vi "ReMiRCAutoCamCalibration.vi"() -> ()   [LabVIEW 2019]
panel:
  in  "stop":bool
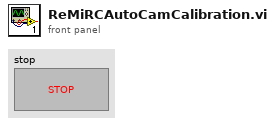
[diagram p1: front panel]
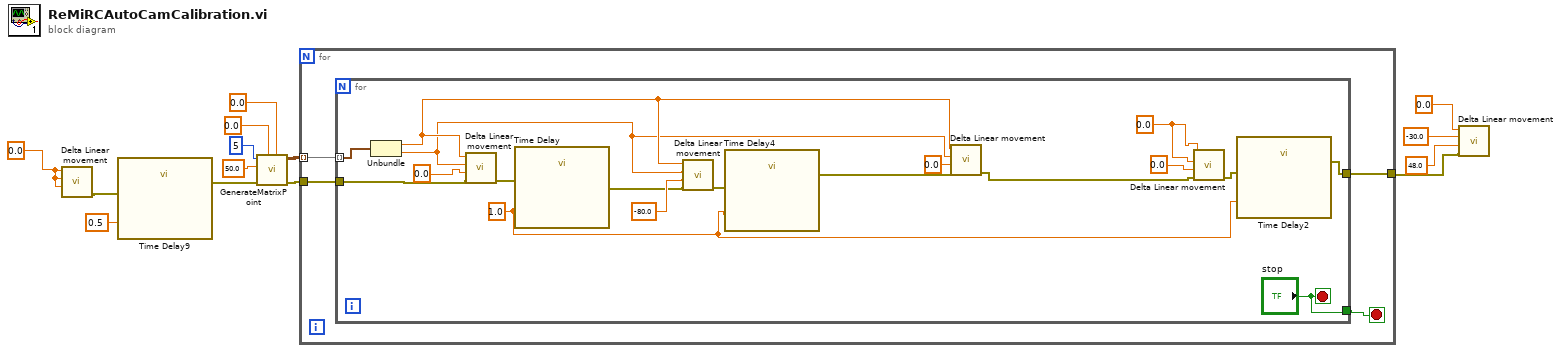
[diagram p0: block diagram]
diagram:
  w6 = 0.0 ("x0")
  n1 = call "Delta Linear movement.vi"("z0"=w6, "y0"=w6, "x0"=w6) -> ("error out"=w5:errorcluster)  [unwired: 8 in]
  n2 = call "Time Delay9"("error in (no error)"=w5, "Delay Time (s)"=0.5) -> ("error out"=w14:errorcluster)  [unwired: 9 in]
  n3 = call "GenerateMatrixPoint.vi"("YOffSet"=0.0, "XOffSet"=0.0, "error in (no error)"=w14, "Pitch"=50.0, "MatrixSize"=5) -> ("error out"=w9:errorcluster, "MatrixPoint"=w8:cluster{dbl, dbl}[][])  [unwired: 5 in]
  n4 = for {
    tunnel: w9 -> [w18]
    tunnel: w8 -> [w16] mode=indexing
    tunnel: [w17] -> w4
    stop <- w15 stop-if-true
    n5 = for {
      tunnel: w18 -> [w25]
      tunnel: [w34] -> w17
      tunnel: w16 -> [w36] mode=indexing
      tunnel: ["stop"] -> w15
      stop <- "stop" stop-if-true
      w35 = 1.0 ("Delay Time (s)")
      w31 = 0.0 ("y0")
      n6 = Unbundle(w36) -> (w21:dbl, w20:dbl)
      n7 = call "Delta Linear movement.vi"("error in (no error)"=w25, "z0"=0.0, "y0"=w20, "x0"=w21) -> ("error out"=w24:errorcluster)  [unwired: 7 in]
      n8 = call "Time Delay"("error in (no error)"=w24, "Delay Time (s)"=w35) -> ("error out"=w28:errorcluster)  [unwired: 9 in]
      n9 = call "Delta Linear movement.vi"("error in (no error)"=w28, "z0"=-80.0, "y0"=w20, "x0"=w21) -> ("error out"=w27:errorcluster)  [unwired: 7 in]
      n10 = call "Time Delay4"("error in (no error)"=w27, "Delay Time (s)"=w35) -> ("error out"=w23:errorcluster)  [unwired: 9 in]
      n11 = call "Delta Linear movement.vi"("error in (no error)"=w23, "z0"=0.0, "y0"=w20, "x0"=w21) -> ("error out"=w22:errorcluster)  [unwired: 7 in]
      n12 = call "Delta Linear movement.vi"("error in (no error)"=w22, "z0"=0.0, "y0"=w31, "x0"=w31) -> ("error out"=w32:errorcluster)  [unwired: 7 in]
      n13 = call "Time Delay2"("error in (no error)"=w32, "Delay Time (s)"=w35) -> ("error out"=w34:errorcluster)  [unwired: 9 in]
    }
  }
  n14 = call "Delta Linear movement.vi"("error in (no error)"=w4, "z0"=48.0, "y0"=-30.0, "x0"=0.0) -> ()  [unwired: 7 in, 1 out]
